vi "CollectICS_alerts.vi"(10 "Prefix":string, 11 "AlertPath":path) -> (2 "Alerts":T1(array[cluster]))   [LabVIEW 2011]
panel:
  out "Numeric":i32
  out "text":string
  out "filenames":string[](array[string])
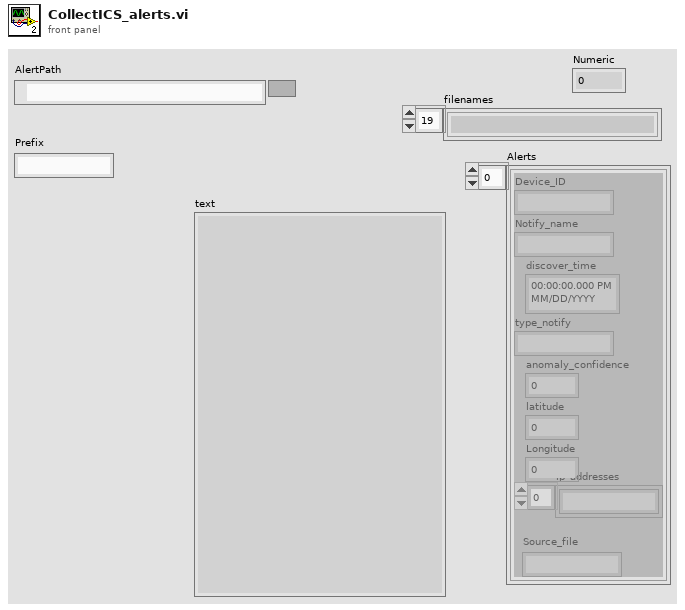
[diagram p1: front panel]
types:
  T1 = cluster{"Device_ID":string, "Notify_name":string, "discover_time":timestamp, "type_notify":string, "anomaly_confidence":dbl, "latitude":dbl, "Longitude":dbl, "ip_addresses":string[], "Source_file":string}[]
  T2 = cluster{"Device_ID":string, "Notify_name":string, "discover_time":timestamp, "type_notify":string, "anomaly_confidence":dbl, "latitude":dbl, "Longitude":dbl, string[], "Source_file":string}[]
  T3 = cluster{"Device_ID":string, "Notify_name":string, "discover_time":timestamp, "type_notify":string, "anomaly_confidence":dbl, "latitude":dbl, "Longitude":dbl, "ip_addresses":string[], "Source_file":string}
  T4 = cluster{"tag_label":string, "tag_value":string}[]
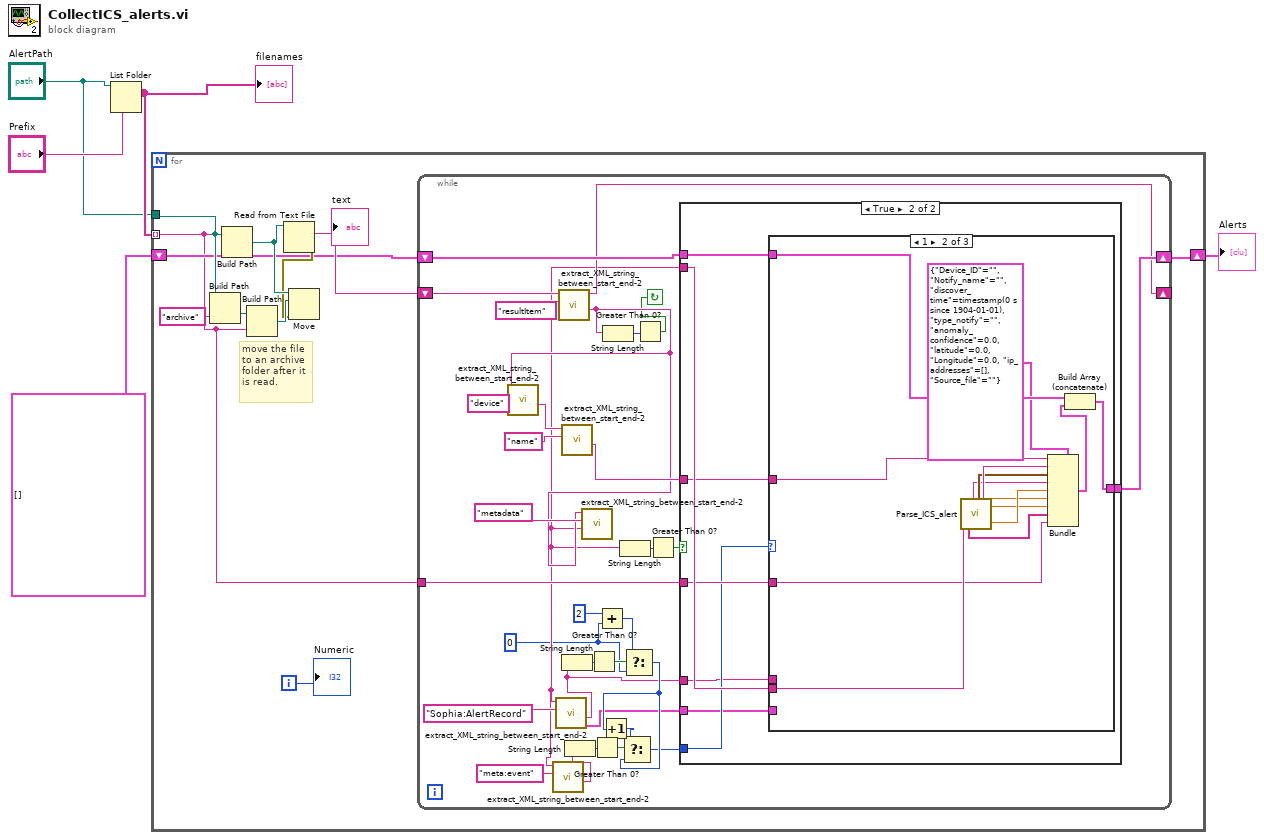
[diagram p0: block diagram]
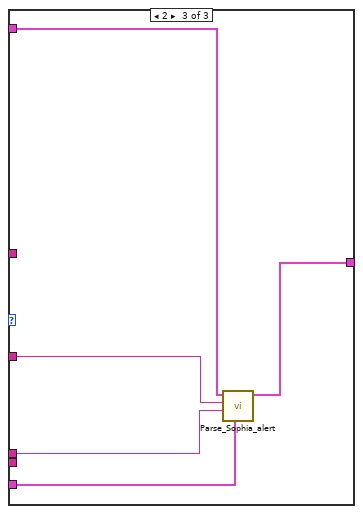
[diagram p4: hidden frame]
diagram:
  n1 = List Folder(path="AlertPath", pattern="Prefix") -> (filenames=w4:string[])  [unwired: 2 in, 3 out]
  "filenames" <- w4
  n2 = for {
    tunnel: w4 -> [w6] mode=indexing
    tunnel: "AlertPath" -> [w13]
    shift-right: [w7] -> w1
    shift-left: T2 [] ("Alerts") -> [w8]
    i -> [w15]
    # "move the file\nto an archive\nfolder after it\nis read."
    n3 = Build Path(base path=w13, name or relative path="archive") -> (appended path=w14:path)
    n4 = Build Path(base path=w13, name or relative path=w6) -> (appended path=w10:path)
    n5 = Build Path(base path=w14, name or relative path=w6) -> (appended path=w11:path)
    n6 = Read from Text File(file (use dialog)=w10) -> (text=w16:string, error out=w9:errorcluster)  [unwired: 3 in, 2 out]
    "text" <- w16
    n7 = Move(source path=w10, error in=w9, 10:w11) -> ()  [unwired: 2 in, 3 out]
    n8 = while {
      shift-right: [w38] -> w7
      shift-left: w8 -> [w39]
      shift-right: [w34] -> _
      shift-left: w16 -> [w48]
      tunnel: w6 -> [w33]
      stop <- w35 continue-if-true
      w25 = 0
      n9 = call "extract_XML_string_between_start_end-2.vi"("type"="resultItem", "XML_Cluster_String in"=w48) -> ("XML_between_startANDEnd"=w37:string, "XML_after_start_end_pair"=w34:string)  [unwired: 6 in, 2 out]
      n10 = call "extract_XML_string_between_start_end-2.vi"("type"="device", "XML_Cluster_String in"=w37) -> ("XML_between_startANDEnd"=w45:string)  [unwired: 6 in, 3 out]
      n11 = call "extract_XML_string_between_start_end-2.vi"("type"="name", "XML_Cluster_String in"=w45) -> ("XML_between_startANDEnd"=w40:string)  [unwired: 6 in, 3 out]
      n12 = call "extract_XML_string_between_start_end-2.vi"("type"="metadata", "XML_Cluster_String in"=w37) -> ("XML_between_startANDEnd"=w30:string)  [unwired: 6 in, 3 out]
      n13 = call "extract_XML_string_between_start_end-2.vi"("type"="meta:event", "XML_Cluster_String in"=w30) -> ("XML_between_startANDEnd"=w27:string)  [unwired: 6 in, 3 out]
      n14 = call "extract_XML_string_between_start_end-2.vi"("type"="Sophia:AlertRecord", "XML_Cluster_String in"=w30) -> ("InTagDefines"=w17:T4, "XML_between_startANDEnd"=w18:string)  [unwired: 6 in, 2 out]
      n15 = String Length(string=w18) -> (length=w29:i32)
      n16 = String Length(string=w27) -> (length=w28:i32)
      n17 = Greater Than 0?(x=w29) -> (x > 0?=w26:bool)
      n18 = Greater Than 0?(x=w28) -> (x > 0?=w22:bool)
      n19 = Add(x=2, y=w25) -> (x+y=w23:i32)
      n20 = String Length(string=w37) -> (length=w36:i32)
      n21 = String Length(string=w30) -> (length=w41:i32)
      n22 = Select(t=w23, s=w26, f=w25) -> (s? t:f=w21:i32)
      n23 = Increment(x=w21) -> (x+1=w20:i32)
      n24 = Select(t=w20, s=w22, f=w21) -> (s? t:f=w19:i32)
      n25 = Greater Than 0?(x=w36) -> (x > 0?=w35:bool)
      n26 = Greater Than 0?(x=w41) -> (x > 0?=w42:bool)
      n27 = case shown="True" w42 {
        tunnel: w30 -> [_ w57]
        tunnel: w40 -> [_ w56]
        tunnel: [w49 w55] -> w38
        tunnel: w39 -> [w49 w54]
        tunnel: w33 -> [_ w53]
        tunnel: w19 -> [_ w52]
        tunnel: w18 -> [_ w51]
        tunnel: w17 -> [_ w50]
        frame False {
        }
        frame True {
          n28 = case shown="1" w52 {
            tunnel: w57 -> [_ w72 _]
            tunnel: w56 -> [_ w71 _]
            tunnel: [w58 w63 w74] -> w55
            tunnel: w54 -> [w58 w61 w73]
            tunnel: w53 -> [_ w60 w76]
            tunnel: w51 -> [_ _ w77]
            tunnel: w50 -> [_ _ w75]
            frame 0, Default {
            }
            frame 1 {
              n29 = call "Parse_ICS_alert.vi"("Meta_data_XML_INLSA"=w72) -> ("Array_of_IPs"=w64:string[], "Numeric"=w67:dbl, "Confidence"=w68:string, "time stamp"=w69:timestamp, "XML_between_startANDEnd 2"=w70:string, "Longitude 2"=w65:dbl, "latitude 2"=w66:dbl)  [unwired: 6 in, 6 out]
              n30 = Bundle(cluster=T3 {"Device_ID"="", "Notify_name"="", "discover_time"=timestamp(0 s since 1904-01-01), "type_notify"="", "anomaly_confidence"=0.0, "latitude"=0.0, "Longitude"=0.0, "ip_addresses"=[], "Source_file"=""}, "Device_ID"=w71, "Notify_name"=w70, "discover_time"=w69, "type_notify"=w68, "anomaly_confidence"=w67, "latitude"=w66, "Longitude"=w65, "ip_addresses"=w64, "Source_file"=w60) -> (w62:T3)
              n31 = Build Array (concatenate)(w61, w62) -> (w63:T1)
            }
            frame 2 {
              n32 = call "Parse_Sophia_alert.vi"("InTagDefines"=w75, "XML_between_startANDEnd"=w77, "source_file_name"=w76, "Alerts_IN"=w73) -> ("Alerts_OUT"=w74:T1)  [unwired: 7 in]
            }
          }
        }
      }
    }
    "Numeric" <- w15
  }
  "Alerts" <- w1
